vi "Assync Lock-in .vi"() -> ()   [LabVIEW 2016]
uses:
  <vilib>/measure/matone.llb/Extract Single Tone Information 1 Chan.vi
  <vilib>/measure/NI_MAPro.lvlib
panel:
  in  "Save result":bool
  out "detected phase (deg)":dbl format="%#_20p"
  out "XY Graph":cluster{dbl[], "Y":dbl[]}[](graph)
  in  "Phase shift":dbl=134.0
  in  "Clip units of Ts off":dbl
  in  "Filter type":enum16{"None", "IIR", "FIR"}(ring)=enum."IIR"
  in  "Fix time delay":bool=TRUE
  in  "Time constant":dbl=0.0001 format="%#_6p"
  out "detected frequency":dbl format="%#_20p"
  out "Waveform Graph":waveform(dbl)[](graph)
  in  "Input file":path
  in  "Reference channel":string="IL2"
  in  "Signal channel":string="VL2"
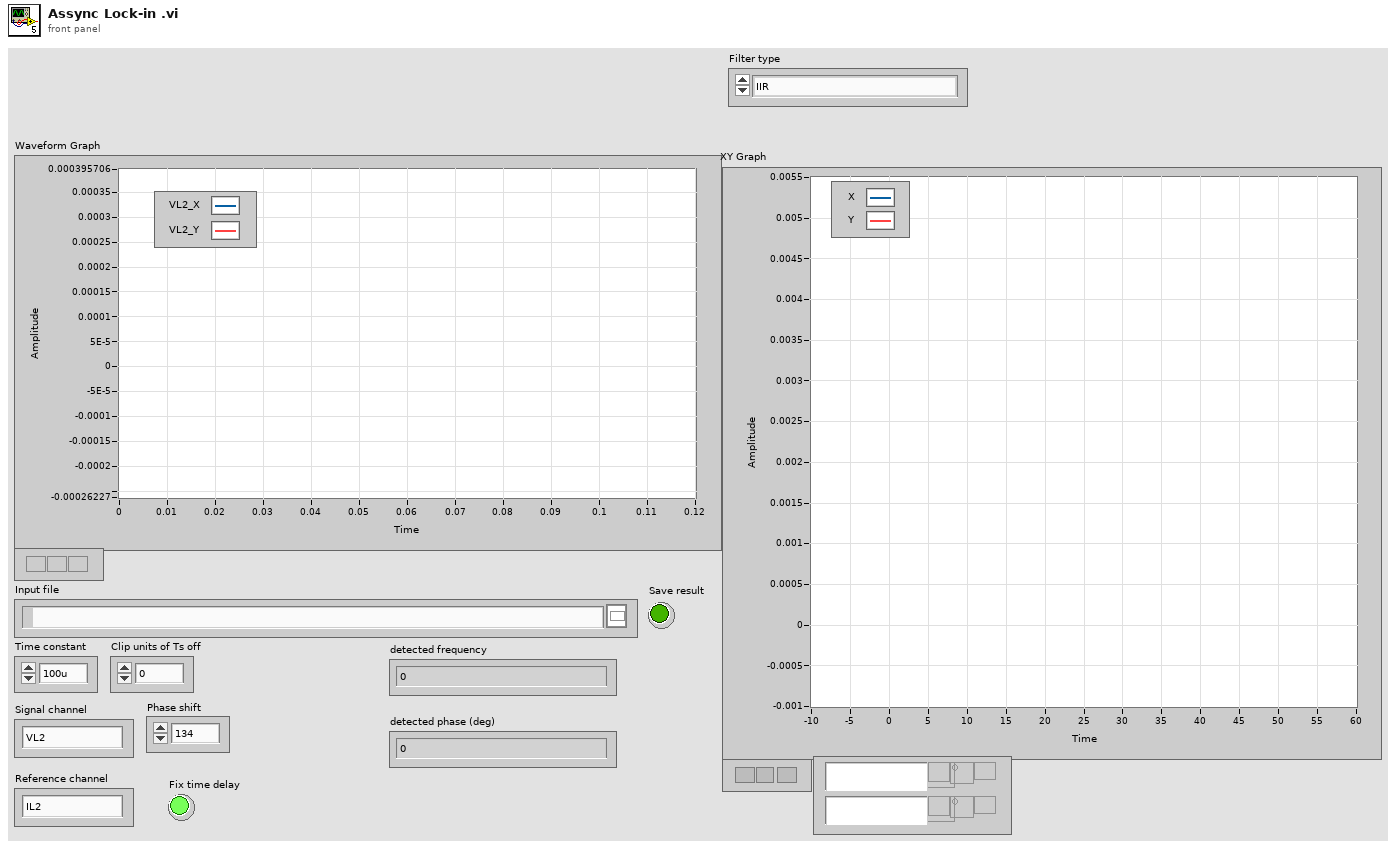
[diagram p1: front panel]
types:
  T1 = enum16{"open", "open or create", "create or replace", "create", "open (read-only)"}
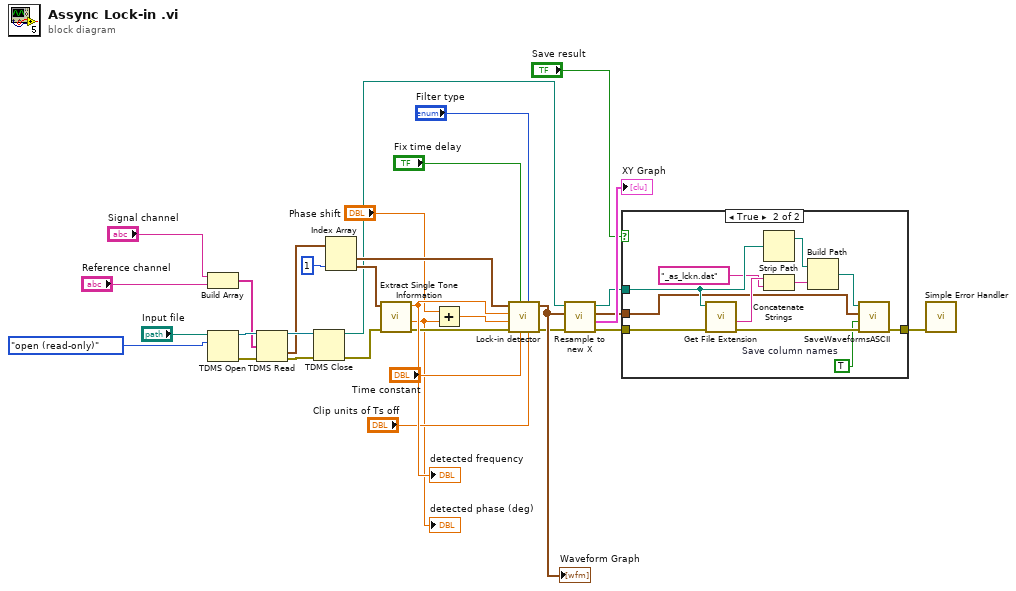
[diagram p0: block diagram]
diagram:
  n1 = Build Array("Signal channel", "Reference channel") -> (w26:string[])
  n2 = TDMS Open(10:T1."open (read-only)" ("operation (0:open)"), 11:"Input file") -> (0:w29:errorcluster, 3:w30:refnum<k34>)  [unwired: 5 in]
  n3 = TDMS Read(0:w30, 7:w26, 11:w29) -> (4:w25:refnum<k34>, 10:w23:waveform(dbl)[], 15:w24:errorcluster)  [unwired: 5 in, 3 out]
  n4 = TDMS Close(8:w24, 11:w25) -> (0:w17:errorcluster, 3:w9:path)
  n5 = Index Array(array=w23, index #2=1 ("index")) -> (element #1=w20:waveform(dbl), element #2=w21:waveform(dbl))  [unwired: 1 in]
  n6 = call-poly <vilib>:"Extract Single Tone Information.vi"("error in (no error)"=w17, "time signal in"=w21) -> ("error out"=w18:errorcluster, "detected phase (deg)"=w6:dbl, "detected frequency"=w19:dbl)  [unwired: 4 in, 3 out]
  "detected frequency" <- w19
  "detected phase (deg)" <- w6
  n7 = Add(x="Phase shift", y=w6) -> (x+y=w12:dbl)
  n8 = call "Lock-in detector.vi"("Clip units of Ts off"="Clip units of Ts off", "Filter type"="Filter type", "Time constant"="Time constant", "Fix time delay"="Fix time delay", "Error In"=w18, "Phase"=w12, "Frequency"=w19, "Data in"=w20) -> ("Error Out"=w8:errorcluster, "Data out"=w10:waveform(dbl)[])  [unwired: 2 in]
  "Waveform Graph" <- w10
  n9 = call "Resample to new X.vi"("Error In"=w8, "Signal"=w10, "X-axis file"=w9) -> ("Error Out"=w3:errorcluster, "XY Graph"=→"XY Graph":cluster{dbl[], "Y":dbl[]}[], "Resampled Signal"=w4:waveform(dbl)[], "X-axis file out"=w5:path)  [unwired: 5 in]
  n10 = case shown="True" "Save result" {
    tunnel: w5 -> [_ w44]
    tunnel: w4 -> [_ w39]
    tunnel: w3 -> [w33 w36]
    tunnel: [w33 w35] -> w1
    frame False {
    }
    frame True {
      w34 = TRUE  # Save column names
      n11 = call <vilib>:"Get File Extension.vi"("error in (no error)"=w36, "file"=w44) -> ("error out"=w37:errorcluster, "filename without extension"=w43:string)  [unwired: 5 in, 3 out]
      n12 = Strip Path(path=w44) -> (stripped path=w41:path)  [unwired: 1 out]
      n13 = Concatenate Strings(w43, "_as_lckn.dat" ("string")) -> (w40:string)
      n14 = Build Path(base path=w41, name or relative path=w40) -> (appended path=w38:path)
      n15 = call "SaveWaveformsASCII.vi"("Error In"=w37, "Save column names"=w34, "Waveforms"=w39, "File"=w38) -> ("Error Out"=w35:errorcluster)  [unwired: 6 in, 1 out]
    }
  }
  n16 = call <vilib>:"Simple Error Handler.vi"("error in (no error)"=w1) -> ()  [unwired: 4 in, 5 out]
